vi "Phase_Av_Weighted_Cross_Moments.vi"(0 "AI Cluster 1":T2={"Colour"=0, "Inst type"=enum."Pitot-static tube", "Inst name"="Manometer voltage", "Symbol"="U", "Code name"="", "Extra Info"="U", "Inst Array"=enum."PWA", "Extra Titles"=[], "Extra Values"=[], "U"=0.0, "u^2"=0.0, "u^3"=0.0, "u^4"=0.0, "Skew_u"=0.0, "Kurt_u"=0.0, "Sd Error in Mean"=0.0, "% u'/U"=0.0, "X"=0.0, "Y"=0.0, "Z"=0.0, "Timescale integral to 25%"=0.0, "Sd Error in Variance"=0.0, "Calib File"=path "", "Calib Constants"=[], "Output Position"=FALSE, "Full Stats"=FALSE, "Av Sampling Rate"=0.0, "Av No of Samples"=0.0, "Total Meas Time (s)"=0.0, "ADAM Ch Name"=""} {"Sd Error in Variance" format="%.2f"; "Skew_u" format="%.2f"; "% u'/U" format="%.2f"; "Sd Error in Mean" format="%.2f"; "Kurt_u" format="%.2f"; "u^4" format="%.2f"; "u^3" format="%.2f"; "U" format="%.2f"; "u^2" format="%.2f"}, 1 "WT Revolution Start times":dbl[](array[numeric]), 5 "Time Cluster 1":T1, 7 "AI Cluster 2":T2={"Colour"=0, "Inst type"=enum."Pitot-static tube", "Inst name"="Manometer voltage", "Symbol"="U", "Code name"="", "Extra Info"="U", "Inst Array"=enum."PWA", "Extra Titles"=[], "Extra Values"=[], "U"=0.0, "u^2"=0.0, "u^3"=0.0, "u^4"=0.0, "Skew_u"=0.0, "Kurt_u"=0.0, "Sd Error in Mean"=0.0, "% u'/U"=0.0, "X"=0.0, "Y"=0.0, "Z"=0.0, "Timescale integral to 25%"=0.0, "Sd Error in Variance"=0.0, "Calib File"=path "", "Calib Constants"=[], "Output Position"=FALSE, "Full Stats"=FALSE, "Av Sampling Rate"=0.0, "Av No of Samples"=0.0, "Total Meas Time (s)"=0.0, "ADAM Ch Name"=""} {"Sd Error in Variance" format="%.2f"; "Skew_u" format="%.2f"; "% u'/U" format="%.2f"; "Sd Error in Mean" format="%.2f"; "Kurt_u" format="%.2f"; "u^4" format="%.2f"; "u^3" format="%.2f"; "U" format="%.2f"; "u^2" format="%.2f"}, 9 "Time Cluster 2":T1, 11 "Shift in":dbl[][](array[numeric]) format="%.2f", 12 "interp. method":i32(ring) items=["nearest", "linear", "spline", "cubic Hermite", "Lagrange"], 13 "No Of Bins":i32) -> (4 "Phase locked uw":dbl[](array[numeric]), 6 "Phase locked uw/u'w'":dbl[](array[numeric]), 15 "Shift out":dbl[][](array[numeric]) format="%.2f")   [LabVIEW 2013]
uses:
  Controls/Analysis_info_cluster.ctl
  Controls/Inst_type.ctl
  Controls/Instrument_Array.ctl
  Controls/Time_Trace_Cluster.ctl
  Globals/Meas_global.vi
panel:
  out "Array":cluster{"Points":dbl[][]}[](array[cluster])
  in  "Time Cluster 3":cluster{"Points":dbl[][]}
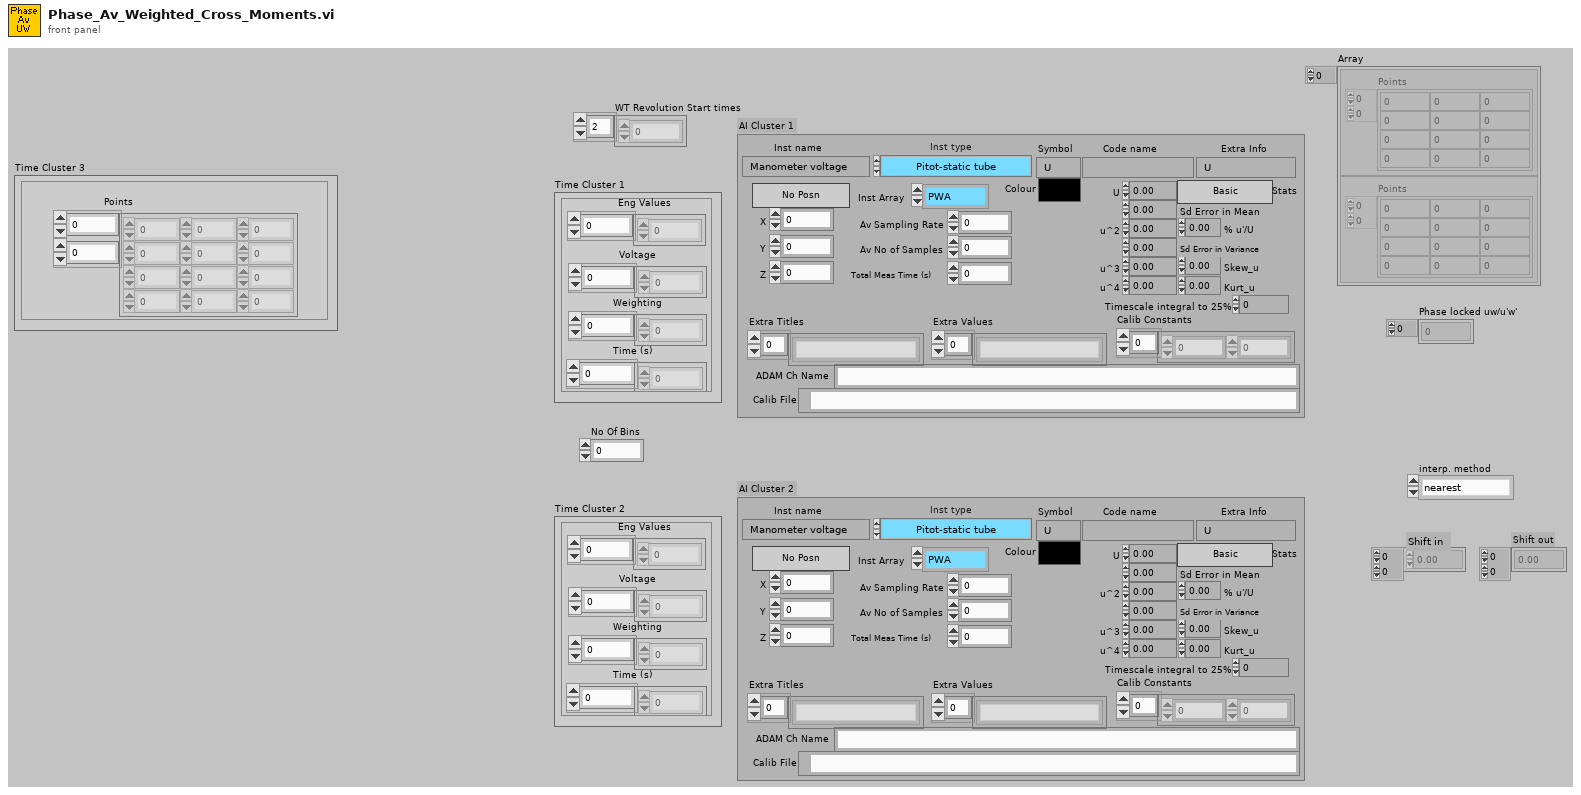
[diagram p1: front panel]
types:
  T1 = typedef "Time_Trace_Cluster.ctl" = cluster{"Weighting":dbl[], "Time (s)":dbl[], "Voltage":dbl[], "Eng Values":dbl[]}
  T2 = typedef "Analysis_info_cluster.ctl" = cluster{"Colour":u32, "Inst type":T3, "Inst name":string, "Symbol":string, "Code name":string, "Extra Info":string, "Inst Array":T4, "Extra Titles":string[], "Extra Values":string[], "U":dbl, "u^2":dbl, "u^3":dbl, "u^4":dbl, "Skew_u":dbl, "Kurt_u":dbl, "Sd Error in Mean":dbl, "% u'/U":dbl, "X":dbl, "Y":dbl, "Z":dbl, "Timescale integral to 25%":dbl, "Sd Error in Variance":dbl, "Calib File":path, "Calib Constants":dbl[], "Output Position":bool, "Full Stats":bool, "Av Sampling Rate":dbl, "Av No of Samples":dbl, "Total Meas Time (s)":dbl, "ADAM Ch Name":string}
  T3 = typedef "Inst_type.ctl" = enum16{"Propeller anemometer", "Raw voltage", "Pressure Transducer", "Pitot-static tube", "Preston tube", "Hot wire", "Cross wire 1", "Cross wire 2", "Generic Linear", "Generic Polynomial", "Generic BackPoly", "Fast FID", "Thermocouple", "Cold wire", "Pulsed Wire", "LDA Vel", "LDA Tran time", "LDA Arr time"}
  T4 = typedef "Instrument_Array.ctl" = enum16{"PWA", "LDA", "Analogue"}
  T5 = typedef "Correlation_cluster1.ctl" = cluster{"U inst":string, "uw":dbl, "u^2w":dbl, "uw^2":dbl, "uw/u'w'":dbl, "W inst":string, "uw^3":dbl, "u^3w":dbl, "u^2w^2":dbl, "Index U":i32, "Index W":i32}
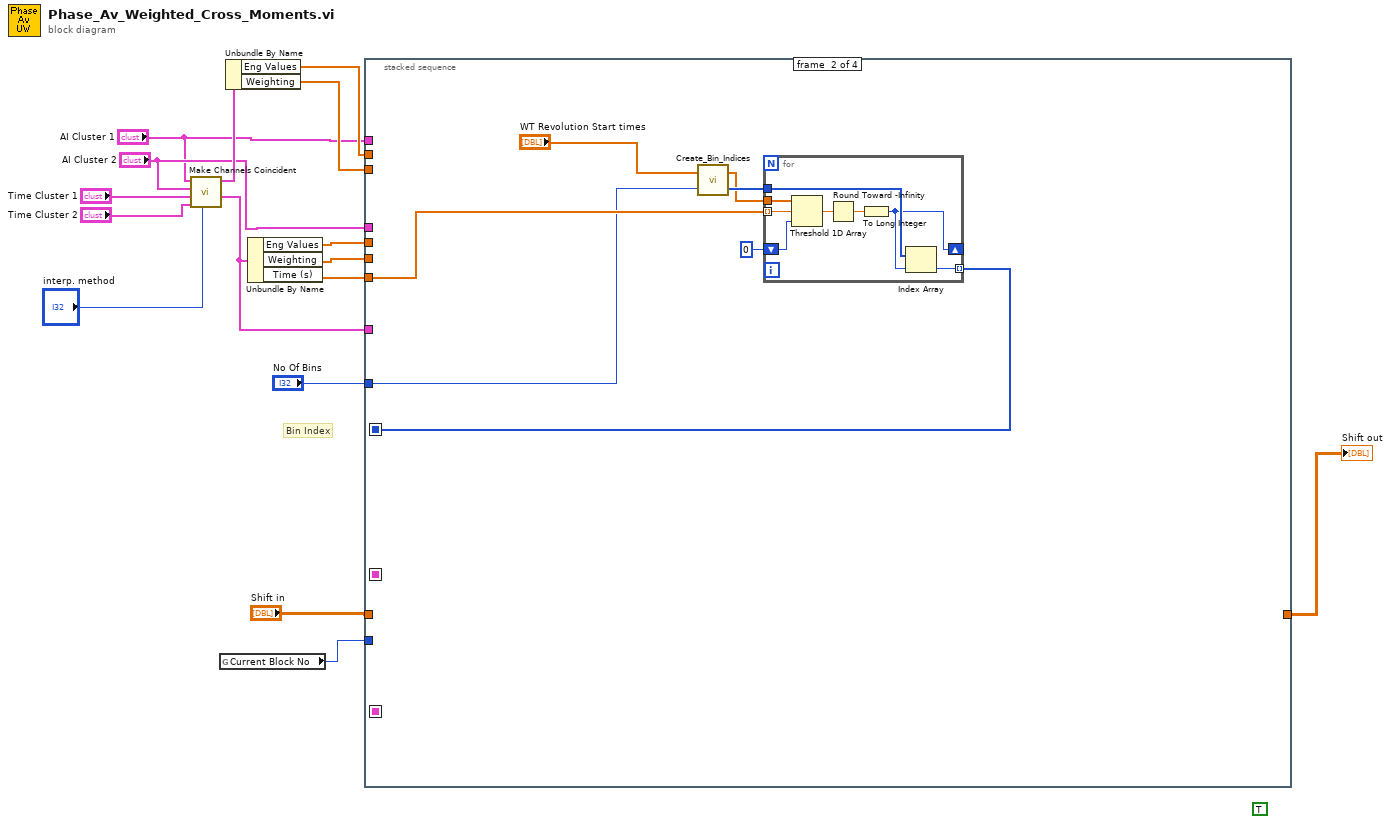
[diagram p0: block diagram]
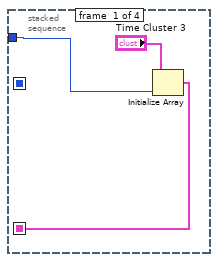
[diagram p2: hidden frame]
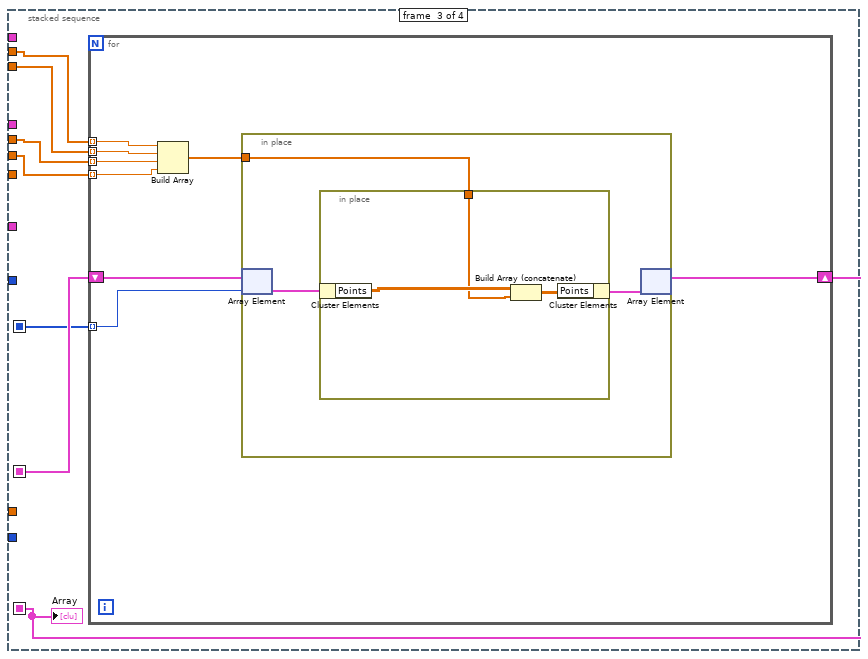
[diagram p3: hidden frame]
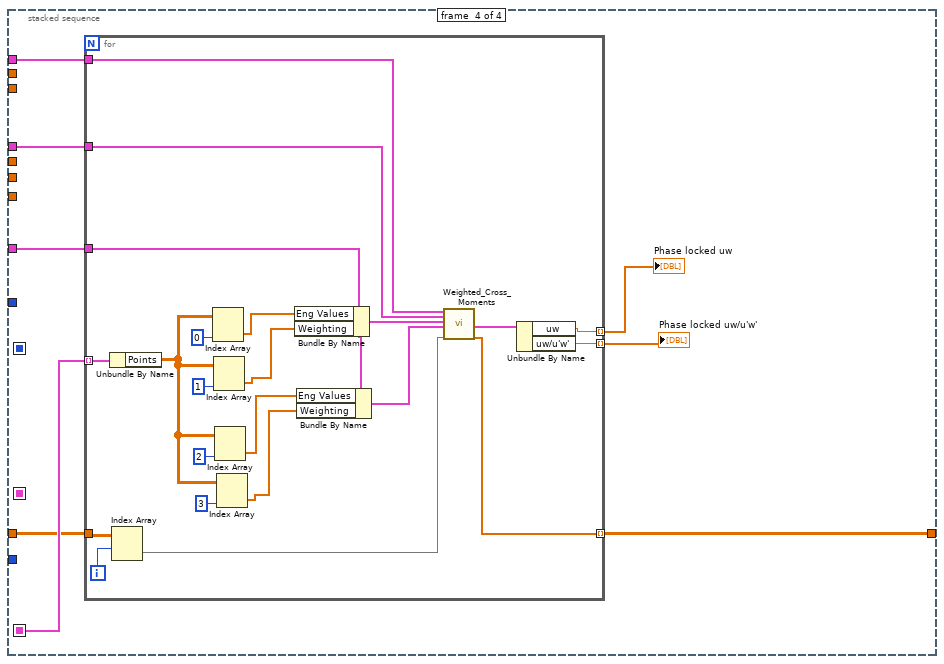
[diagram p4: hidden frame]
diagram:
  (unwired) TRUE
  # "Bin Index"
  n1 = call "Make Channels Coincident.vi"("interp. method"="interp. method", "Time Cluster 2"="Time Cluster 2", "Time Cluster 1"="Time Cluster 1", "Cluster 2"="AI Cluster 2", "Cluster 1"="AI Cluster 1") -> ("Coincident Time Cluster 2"=w5:T1, "Coincident Time Cluster 1"=w6:T1)  [unwired: 5 in]
  n2 = global read "Meas_global.vi" "Current Block No"() -> (w16:i32)
  n3 = Unbundle By Name(w6) -> ("Eng Values"=w13:dbl[], "Weighting"=w12:dbl[])
  n4 = Unbundle By Name(w5) -> ("Eng Values"=w11:dbl[], "Weighting"=w10:dbl[], "Time (s)"=w4:dbl[])
  n5 = stacked-sequence {
    seq-local: [_ w21 _ _] -> [_ _ w40 _]
    seq-local: [w17 _ _ _] -> [_ _ w41 _]
    seq-local: [_ _ w35 _] -> [_ _ _ w62]
    tunnel: w13 -> [_ _ w39 _]
    tunnel: "Shift in" -> [_ _ _ w59]
    tunnel: w11 -> [_ _ w37 _]
    tunnel: w16 -> [_ _ _ _]
    tunnel: w12 -> [_ _ w38 _]
    tunnel: w10 -> [_ _ w36 _]
    tunnel: "AI Cluster 1" -> [_ _ _ w61]
    tunnel: "AI Cluster 2" -> [_ _ _ w60]
    tunnel: [_ _ _ w58] -> w15
    tunnel: w5 -> [_ _ _ w63]
    tunnel: w4 -> [_ w22 _ _]
    tunnel: "No Of Bins" -> [w19 w20 _ _]
    frame #0 {
      n6 = Initialize Array("Time Cluster 3", w19) -> (w17:cluster{"Points":dbl[][]}[])
    }
    frame #1 {
      n7 = call "Create_Bin_Indices.vi"("No Of Bins"=w20, "Cycle Start TIme"="WT Revolution Start times") -> ("Bin Number"=w26:i32[], "Bin Start Time"=w25:dbl[])
      n8 = for {
        tunnel: w25 -> [w34]
        tunnel: w22 -> [w33] mode=indexing
        shift-right: [w30] -> _
        shift-left: 0 -> [w27]
        tunnel: w26 -> [w31]
        tunnel: [w29] -> w21 mode=indexing
        n9 = Threshold 1D Array(1:w27, 2:w33, 3:w34) -> (0:w32:dbl)
        n10 = Round Toward -Infinity(1:w32) -> (0:w28:dbl)
        n11 = To Long Integer(number=w28) -> (32bit integer=w30:i32)
        n12 = Index Array(array=w31, index=w30) -> (element=w29:i32)
      }
    }
    frame #2 {
      n13 = for {
        shift-right: [w47] -> w35
        shift-left: w41 -> [w48]
        tunnel: w40 -> [w49] mode=indexing
        tunnel: w39 -> [w46] mode=indexing
        tunnel: w38 -> [w45] mode=indexing
        tunnel: w37 -> [w44] mode=indexing
        tunnel: w36 -> [w43] mode=indexing
        n14 = Build Array(w46, w45, w44, w43) -> (w42:dbl[])
        n15 = in-place {
          in-place-border: w42 -> [w50]
          n16 = in-place-array #1(w48, w49) -> (w52:cluster{"Points":dbl[][]})
          n17 = in-place {
            in-place-border: w50 -> [w54]
            n18 = in-place-cluster #2(w52) -> ("Points"=w55:dbl[][])
            n19 = Build Array (concatenate)(w55, w54) -> (w53:dbl[][])
            n20 = in-place-cluster #2("Points"=w53) -> (w51:cluster{"Points":dbl[][]})
          }
          n21 = in-place-array #1(w51) -> (w47:cluster{"Points":dbl[][]}[])  [unwired: 1 out]
        }
      }
      "Array" <- w35
    }
    frame #3 {
      n22 = for {
        tunnel: w63 -> [w85]
        tunnel: w62 -> [w84] mode=indexing
        tunnel: w61 -> [w74]
        tunnel: w60 -> [w73]
        tunnel: w59 -> [w68]
        tunnel: [w70] -> w58 mode=indexing
        tunnel: [w65] -> w57 mode=indexing
        tunnel: [w64] -> w56 mode=indexing
        i -> [w69]
        n23 = Unbundle By Name(w84) -> ("Points"=w78:dbl[][])
        n24 = Index Array(array=w68, index (row)=w69) -> (element=w67:dbl[])  [unwired: 1 in]
        n25 = Index Array(array=w78, index (col)=0 ("disabled index (col)")) -> (element=w82:dbl[])  [unwired: 1 in]
        n26 = Index Array(array=w78, index (col)=1 ("disabled index (col)")) -> (element=w75:dbl[])  [unwired: 1 in]
        n27 = Index Array(array=w78, index (col)=2 ("disabled index (col)")) -> (element=w77:dbl[])  [unwired: 1 in]
        n28 = Index Array(array=w78, index (col)=3 ("disabled index (col)")) -> (element=w76:dbl[])  [unwired: 1 in]
        n29 = Bundle By Name(cluster=w85, "Eng Values"=w82, "Weighting"=w75) -> (w72:T1)
        n30 = Bundle By Name(cluster=w85, "Eng Values"=w77, "Weighting"=w76) -> (w71:T1)
        n31 = call "Weighted_Cross_Moments.vi"("AI Cluster 1"=w74, "AI Cluster 2"=w73, "Time Cluster 1"=w72, "Time Cluster 2"=w71, "Shift in"=w67) -> ("output cluster"=w66:T5, "Shift out"=w70:dbl[])  [unwired: 13 in]
        n32 = Unbundle By Name(w66) -> ("uw"=w65:dbl, "uw/u'w'"=w64:dbl)
      }
      "Phase locked uw" <- w57
      "Phase locked uw/u'w'" <- w56
    }
  }
  "Shift out" <- w15
